vi "Read Discrete Inputs1.vi"(8 "error in (no error)":errorcluster, 9 "number of inputs":u16, 10 "starting address":u16, 11 "device data model in":refnum<class "Standard Data Model1.lvclass">) -> (0 "error out":errorcluster, 2 "data":bool[](array[boolean]), 3 "device data model out":refnum<class "Standard Data Model1.lvclass">)   [LabVIEW 2021, in "NI_modbus_upd.lvlib" / "Standard Data Model1.lvclass"]
doc: "Reads N discrete inputs from the data model starting at address M."
uses:
  Standard Data Model1.lvclass
  Standard Data Model1.lvclass/Standard Data Model1.ctl
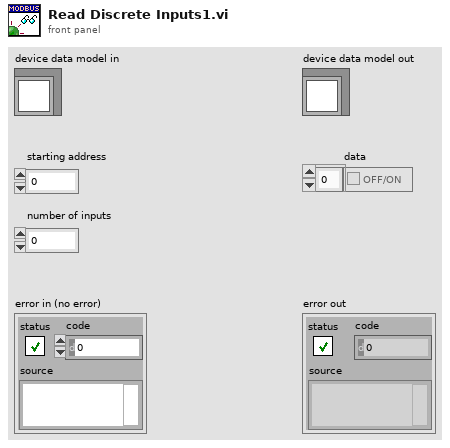
[diagram p1: front panel]
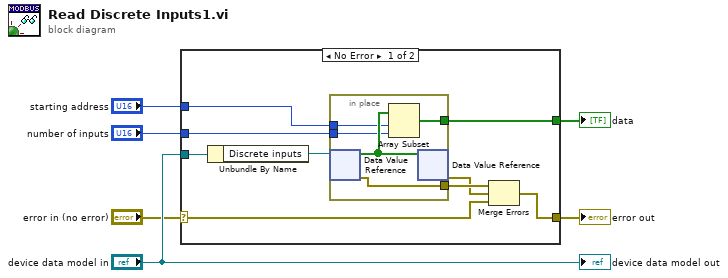
[diagram p0: block diagram]
diagram:
  n1 = case shown="No Error" "error in (no error)" {
    selector: "error in (no error)" -> [w8 w21]
    tunnel: "device data model in" -> [w15 _]
    tunnel: [w14 w21] -> w5
    tunnel: "starting address" -> [w12 _]
    tunnel: "number of inputs" -> [w11 _]
    tunnel: [w10 _] -> w2
    frame No Error {
      n2 = Unbundle By Name(w15) -> ("Discrete inputs"=w13:refnum<data-value>)
      n3 = in-place {
        in-place-border: w12 -> [w19]
        in-place-border: w11 -> [w18]
        in-place-border: [w17] -> w10
        in-place-border: [w16] -> w9
        n4 = in-place-dvr #1(w13) -> (w20:bool[], w16:errorcluster)
        n5 = Array Subset(array=w20, index=w19, length=w18) -> (w17:bool[])
        n6 = in-place-dvr #1(w20) -> (w7:errorcluster)  [unwired: 1 out]
      }
      n7 = Merge Errors(w9, w7, w8) -> (w14:errorcluster)
    }
    frame Error {
    }
  }
  "error out" <- w5
  "data" <- w2
  "device data model out" <- "device data model in"
